vi "Initialize Pod.vi"() -> (0 "error out":errorcluster, 3 "FPGA VI Reference Out":refnum<k20>)   [LabVIEW 2017]
uses:
  <vilib>/FPGAPlugInAG/cRIO-9035 (Sync)/niLvFpga_Open_cRIO-9035 (Sync).vi
  <vilib>/rvi/interface/common/dynamic/niFpgaDynamicAddResources.vi
  <vilib>/rvi/interface/nirviOpenFPGA/nirviOpenFPGA.xnode
  FPGA Bitfiles/Pod2_FPGATarget_FPGA_AwN3-44bkoY.lvbitx
  FPGA.vi
  <vilib>/NI_Real-Time Target Support.lvlib
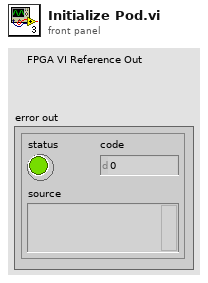
[diagram p1: front panel]
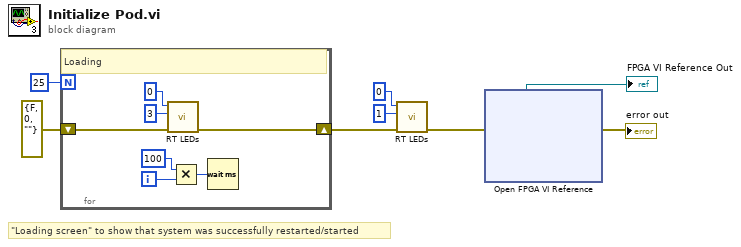
[diagram p0: block diagram]
diagram:
  # "\"Loading screen\" to show that system was successfully restarted/started"
  n1 = for {
    N: 25 -> [_]
    shift-right: [w12] -> w2
    shift-left: errorcluster {"status"=FALSE, "code"=0, "source"=""} ("error out") -> [w15]
    i -> [w11]
    # "Loading"
    n2 = call <vilib>:"RT LEDs.vi"("error in (no error)"=w15, "State"=3, "LED Num"=0) -> ("error out"=w12:errorcluster)  [unwired: 3 in, 1 out]
    n3 = Multiply(x=100, y=w11) -> (x*y=w9:i32)
    n4 = Wait (ms)(milliseconds to wait=w9) -> ()  [unwired: 1 out]
  }
  n5 = call <vilib>:"RT LEDs.vi"("error in (no error)"=w2, "State"=1, "LED Num"=0) -> ("error out"=w1:errorcluster)  [unwired: 3 in, 1 out]
  n6 = xnode "Open FPGA VI Reference"("error in"=w1) -> ("FPGA VI Reference Out"=→"FPGA VI Reference Out":refnum<k20>, "error out"=→"error out":errorcluster)  [unwired: 1 in]
